vi "FindUnexpectedDepsOfLibraries.vi"(6 "Failures Indicator Ref":refnum<vi>, 8 "error in (no error)":errorcluster, 9 "Status Indicator Ref":refnum<vi>, 10 "Lvlib/Lvclass paths":path[](array[path]), 11 "CLI in":refnum<class "CLI.lvclass">) -> (0 "error out":errorcluster, 2 "Failures Array":T1[](array[typedef]), 3 "CLI out":refnum<class "CLI.lvclass">)   [LabVIEW 2019, in "DepsWatch.lvlib"]
uses:
  DepsWatch.lvlib
  Typedefs/DepsCheckResult.ctl
  <vilib>/Wiresmith Technology/G CLI/CLI Class/CLI.lvclass
  <vilib>/Utility/config.llb/NI_LVConfig.lvlib
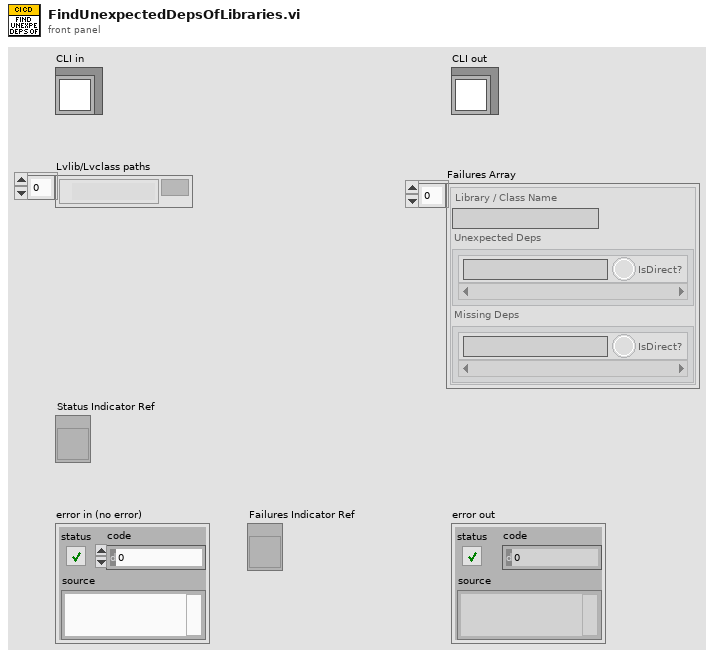
[diagram p1: front panel]
types:
  T1 = typedef "DepsWatch.lvlib/DepsCheckResult.ctl" = cluster{"Library / Class Name":string, "Unexpected Deps":cluster{"Dependency":string, "IsDirect?":bool}[], "Missing Deps":cluster{"Dependency":string, "IsDirect?":bool}[]}
  T2 = typedef "NI_LVConfig.lvlib/Config Data RefNum.ctl" = refnum<k1>
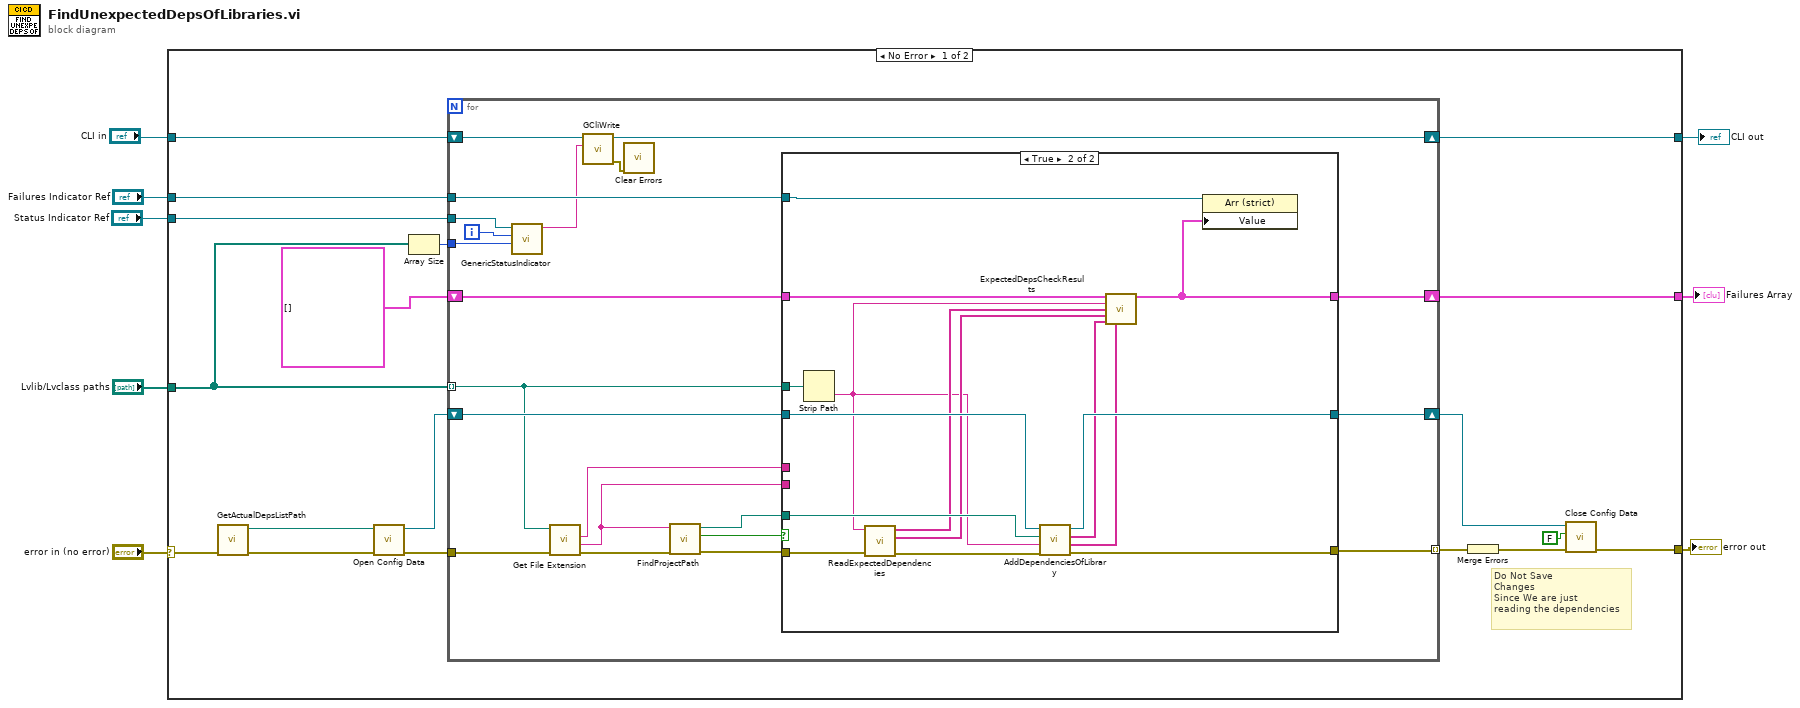
[diagram p0: block diagram]
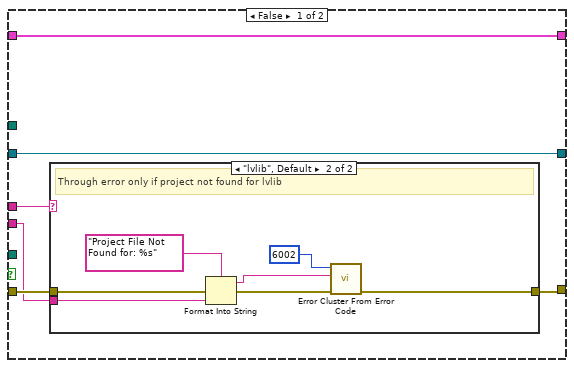
[diagram p2: hidden frame]
diagram:
  n1 = case shown="No Error" "error in (no error)" {
    selector: "error in (no error)" -> [w9 w78]
    tunnel: "Failures Indicator Ref" -> [w26 _]
    tunnel: "Status Indicator Ref" -> [w25 _]
    tunnel: [w24 _] -> w6
    tunnel: [w23 w77] -> w5
    tunnel: [w22 w78] -> w4
    tunnel: "CLI in" -> [w21 w77]
    tunnel: "Lvlib/Lvclass paths" -> [w15 _]
    frame No Error {
      # "Do Not Save\nChanges\nSince We are just\nreading the dependencies"
      n2 = call "GetActualDepsListPath.vi"("error in (no error)"=w9) -> ("error out"=w20:errorcluster, "ActualDepsListPath"=w19:path)  [unwired: 9 in]
      n3 = call <vilib>:"Open Config Data.vi"("error in (no error)"=w20, "configuration file path"=w19) -> ("error out"=w10:errorcluster, "refnum"=w12:T2)  [unwired: 7 in, 1 out]
      n4 = Array Size(array=w15) -> (size(s)=w16:i32)
      n5 = for {
        tunnel: w10 -> [w47]
        tunnel: w15 -> [w27] mode=indexing
        tunnel: [w31] -> w11 mode=indexing
        shift-right: [w41] -> w14
        shift-left: w12 -> [w42]
        tunnel: w16 -> [w40]
        shift-right: [w37] -> w24
        shift-left: T1[] [] -> [w38]
        shift-right: [w36] -> w23
        shift-left: w21 -> [w33]
        tunnel: w25 -> [w35]
        tunnel: w26 -> [w34]
        i -> [w39]
        n6 = call "GenericStatusIndicator.vi"("Total"=w40, "Current Iteration"=w39, "Status Indicator Ref In"=w35) -> ("CLI Status to Print"=w32:string)  [unwired: 8 in]
        n7 = call <vilib>:"Get File Extension.vi"("error in (no error)"=w47, "file"=w27) -> ("error out"=w46:errorcluster, "filename without extension"=w29:string, "lowercase file extension"=w28:string)  [unwired: 5 in, 2 out]
        n8 = call "GCliWrite.vi"("Text to Write"=w32, "CLI in"=w33) -> ("error out"=w30:errorcluster, "CLI out"=w36:refnum<class "CLI.lvclass">)  [unwired: 8 in]
        n9 = call <vilib>:"Clear Errors.vi"("error in (no error)"=w30) -> ()  [unwired: 5 in, 2 out]
        n10 = call "FindProjectPath.vi"("error in (no error)"=w46, "Library/Class Name"=w29) -> ("error out"=w44:errorcluster, "Found?"=w45:bool, "Project Path"=w43:path)  [unwired: 7 in]
        n11 = case shown="True" w45 {
          tunnel: w44 -> [w50 w73]
          tunnel: [w51 w71] -> w31
          tunnel: w43 -> [_ w76]
          tunnel: w42 -> [w53 w75]
          tunnel: [w53 w74] -> w41
          tunnel: w29 -> [w49 _]
          tunnel: w38 -> [w52 w70]
          tunnel: [w52 w68] -> w37
          tunnel: w34 -> [_ w67]
          tunnel: w28 -> [w48 _]
          tunnel: w27 -> [_ w66]
          frame False {
            n12 = case shown="\"lvlib\", Default" w48 {
              tunnel: [w54 w61] -> w51
              tunnel: w50 -> [w54 w59]
              tunnel: w49 -> [_ w57]
              frame "lvclass" {
                # "Skipped when project not found for lvclass."
              }
              frame "lvlib", Default {
                # "Through error only if project not found for lvlib"
                n13 = Format Into String(format string="Project File Not Found for: %s", error in=w59, w57) -> (resulting string=w56:string, error out=w55:errorcluster)  [unwired: 1 in]
                n14 = call <vilib>:"Error Cluster From Error Code.vi"("error in (no error)"=w55, "error message (\"\")"=w56, "error code (0)"=6002) -> ("error out"=w61:errorcluster)  [unwired: 6 in]
              }
            }
          }
          frame True {
            n15 = Strip Path(path=w66) -> (name=w62:string)  [unwired: 1 out]
            n16 = call "ReadExpectedDependencies.vi"("error in (no error)"=w73, "Library Name"=w62) -> ("error out"=w72:errorcluster, "Expected Indirect Dependencies"=w64:string[], "Expected Direct Dependencies"=w69:string[])  [unwired: 5 in, 2 out]
            n17 = call "AddDependenciesOfLibrary.vi"("error in (no error)"=w72, "LibraryName"=w62, "Project Path"=w76, "Config Refnum in"=w75) -> ("error out"=w71:errorcluster, "Indirect ActualDependencies"=w63:string[], "Direct ActualDependencies"=w65:string[], "Config Refnum out"=w74:T2)  [unwired: 4 in]
            n18 = call "ExpectedDepsCheckResults.vi"("ResultsArray"=w70, "Library Name"=w62, "Expected Direct Dependencies"=w69, "Expected Indirect Dependencies"=w64, "Actual Direct Dependencies"=w65, "Actual Indirect Dependencies"=w63) -> ("ResultsArray out"=w68:T1[])  [unwired: 9 in]
            n19 = property class="Arr (strict)"(reference=w67, "Value"=w68) -> ()  [unwired: 1 in, 2 out]
          }
        }
      }
      n20 = Merge Errors(w11) -> (w13:errorcluster)
      n21 = call <vilib>:"Close Config Data.vi"("error in (no error)"=w13, "write file if changed (T)"=FALSE, "refnum"=w14) -> ("error out"=w22:errorcluster)  [unwired: 7 in, 1 out]
    }
    frame Error {
    }
  }
  "Failures Array" <- w6
  "CLI out" <- w5
  "error out" <- w4
